vi "String to TOD Byte Stream.vi"(8 "error in (no error)":errorcluster, 10 "Value":string) -> (0 "error out":errorcluster, 2 "Byte Stream":u8[](array[numeric]))   [LabVIEW 2018, in "TwinCAT ADS.lvclass"]
uses:
  TwinCAT ADS.lvclass
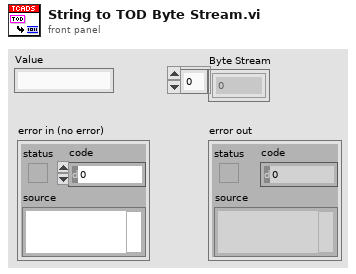
[diagram p1: front panel]
types:
  T1 = enum16{"big-endian, network order", "native, host order", "little-endian"}
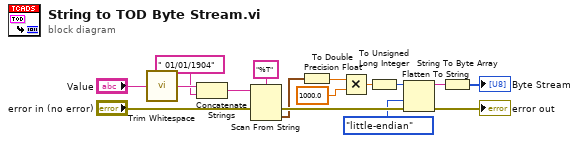
[diagram p0: block diagram]
diagram:
  n1 = call <vilib>:"Trim Whitespace.vi"("string"="Value") -> ("trimmed string"=w8:string)  [unwired: 1 in]
  n2 = Concatenate Strings(w8, " 01/01/1904") -> (w7:string)
  n3 = Scan From String(format string="%T", input string=w7, error in="error in (no error)") -> (error out=w16:errorcluster, output 1=w1:timestamp)  [unwired: 2 in, 2 out]
  n4 = To Double Precision Float(number=w1) -> (double precision float=w14:dbl)
  n5 = Multiply(x=w14, y=1000.0) -> (x*y=w9:dbl)
  n6 = To Unsigned Long Integer(number=w9) -> (unsigned 32bit integer=w12:u32)
  n7 = Flatten To String(anything=w12, byte order (0:big-endian, network order)=T1."little-endian", error in (no error)=w16) -> (data string=w10:string, error out=→"error out":errorcluster)  [unwired: 1 in, 1 out]
  n8 = String To Byte Array(string=w10) -> (unsigned byte array=→"Byte Stream":u8[])
